vi "config_file(SubVI).vi"(9 "all ref":refnum<vi>[](array[refnum]), 10 "文件抬头":string, 11 "文件夹名称":string) -> (3 "字符串输出":string)   [LabVIEW 2019, in "SubVI.lvlib"]
uses:
  SubVI.lvlib
  <vilib>/Utility/Data Type/NI_Data Type.lvlib
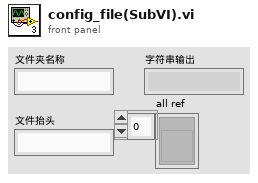
[diagram p1: front panel]
types:
  T1 = enum16{"open", "replace", "create", "open or create", "replace or create", "replace or create with confirmation"}
  T2 = typedef "NI_Data Type.lvlib/Data Type.ctl" = enum8{"Invalid Type", "Void", "I8", "I16", "I32", "I64", "U8", "U16", "U32", "U64", "Single Float", "Double Float", "Extended Float", "Single Complex", "Double Complex", "Extended Complex", "Enum U8", "Enum U16", "Enum U32", "Enum U64", "Single Float With Unit", "Double Float With Unit", "Extended Float With Unit", "Single Complex with Unit", "Double Complex with Unit", "Extended Complex with Unit", "Boolean", "String", "Path", "Picture", "Tag", "Array", "Cluster", "Variant", "LV Variant", "Waveform", "Timestamp", "Digital Waveform", "Digital Data", "ExpressData", "Refnum", "External Data", "VI", "Poly VI", "LabVIEW Class Instance", "Fixed Point", "Set Collection", "Map Collection"}
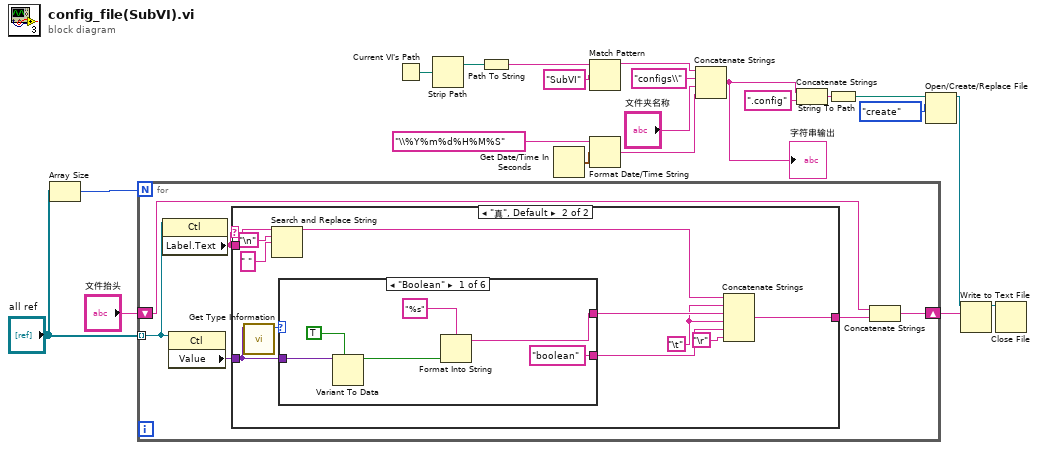
[diagram p0: block diagram]
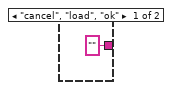
[diagram p2: hidden frame]
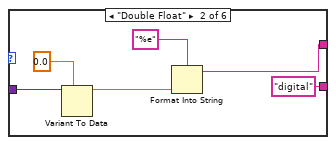
[diagram p3: hidden frame]
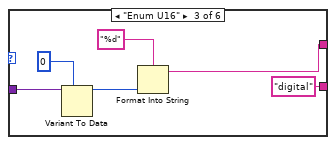
[diagram p4: hidden frame]
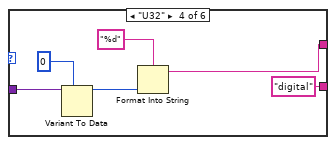
[diagram p5: hidden frame]
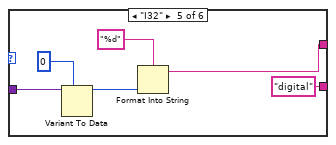
[diagram p6: hidden frame]
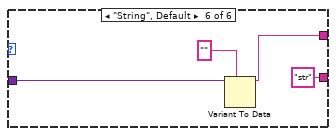
[diagram p7: hidden frame]
diagram:
  n1 = Array Size(array="all ref") -> (size(s)=w8:i32)
  n2 = for {
    N: w8 -> [_]
    shift-right: [w27] -> w15
    shift-left: "文件抬头" -> [w26]
    tunnel: "all ref" -> [w24] mode=indexing
    n3 = property class="Ctl"(reference=w24) -> ("Label.Text"=w23:string)  [unwired: 1 in, 2 out]
    n4 = property class="Ctl"(reference=w24) -> ("Value"=w22:variant)  [unwired: 1 in, 2 out]
    n5 = case shown="\"真\", Default" w23 {
      tunnel: ["" w37] -> w25
      tunnel: w22 -> [_ w30]
      tunnel: w23 -> [_ w29]
      frame "cancel", "load", "ok" {
      }
      frame "真", Default {
        w32 = "\t"
        n6 = call <vilib>:"Get Type Information.vi"("variant"=w30) -> ("type"=w36:T2)  [unwired: 6 in, 4 out]
        n7 = Search and Replace String(input string=w29, search string="\n", replace string=" " ("替换字符串(\"\")")) -> (result string=w35:string)  [unwired: 5 in, 3 out]
        n8 = case shown="\"Boolean\"" w36 {
          tunnel: w30 -> [w45 w51 w57 w63 w69 w73]
          tunnel: [w41 w48 w54 w60 w66 w71] -> w39
          tunnel: ["boolean" "digital" "digital" "digital" "digital" "str"] -> w31
          frame "Boolean" {
            n9 = Variant To Data(type=TRUE, Variant=w45) -> (data=w43:bool)  [unwired: 1 in, 1 out]
            n10 = Format Into String(format string="%s" ("格式字符串"), w43) -> (resulting string=w41:string)  [unwired: 2 in, 1 out]
          }
          frame "Double Float" {
            n11 = Variant To Data(type=0.0, Variant=w51) -> (data=w50:dbl)  [unwired: 1 in, 1 out]
            n12 = Format Into String(format string="%e" ("格式字符串"), w50) -> (resulting string=w48:string)  [unwired: 2 in, 1 out]
          }
          frame "Enum U16" {
            n13 = Variant To Data(type=0, Variant=w57) -> (data=w56:i32)  [unwired: 1 in, 1 out]
            n14 = Format Into String(format string="%d" ("格式字符串"), w56) -> (resulting string=w54:string)  [unwired: 2 in, 1 out]
          }
          frame "U32" {
            n15 = Variant To Data(type=0, Variant=w63) -> (data=w62:i32)  [unwired: 1 in, 1 out]
            n16 = Format Into String(format string="%d" ("格式字符串"), w62) -> (resulting string=w60:string)  [unwired: 2 in, 1 out]
          }
          frame "I32" {
            n17 = Variant To Data(type=0, Variant=w69) -> (data=w68:i32)  [unwired: 1 in, 1 out]
            n18 = Format Into String(format string="%d" ("格式字符串"), w68) -> (resulting string=w66:string)  [unwired: 2 in, 1 out]
          }
          frame "String", Default {
            n19 = Variant To Data(type="", Variant=w73) -> (data=w71:string)  [unwired: 1 in, 1 out]
          }
        }
        n20 = Concatenate Strings(w35, w32, w39, w32, w31, "\r") -> (w37:string)
      }
    }
    n21 = Concatenate Strings(w26, w25) -> (w27:string)
  }
  n22 = Current VI's Path() -> (path=w10:path)
  n23 = Strip Path(path=w10) -> (stripped path=w19:path)  [unwired: 1 out]
  n24 = Path To String(path=w19) -> (string=w7:string)
  n25 = Get Date/Time In Seconds() -> (seconds since 1Jan1904=w12:timestamp)
  n26 = Match Pattern(string=w7, regular expression="SubVI" ("正则表达式")) -> (before substring=w5:string)  [unwired: 1 in, 3 out]
  n27 = Format Date/Time String(time format string (%c)="\\%Y%m%d%H%M%S", seconds (now)=w12) -> (date/time string=w11:string)  [unwired: 1 in]
  n28 = Concatenate Strings(w5, "configs\\" ("字符串"), "文件夹名称", w11) -> (w1:string)
  "字符串输出" <- w1
  n29 = Concatenate Strings(w1, ".config" ("string")) -> (w2:string)
  n30 = String To Path(string=w2) -> (path=w20:path)
  n31 = Open/Create/Replace File(file path (use dialog)=w20, operation (0:open)=T1."create" ("操作(0:open)")) -> (refnum out=w14:refnum<file>)  [unwired: 4 in, 2 out]
  n32 = Write to Text File(file (use dialog)=w14, text=w15) -> (refnum out=w16:refnum<file>)  [unwired: 2 in, 2 out]
  n33 = Close File(refnum=w16) -> ()  [unwired: 1 in, 2 out]
